vi "dioda.vi"() -> ()   [LabVIEW 2012]
panel:
  in  "data":bool[](array[boolean])
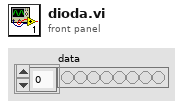
[diagram p1: front panel]
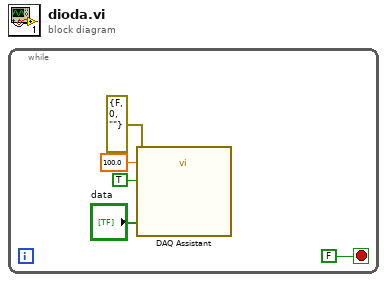
[diagram p0: block diagram]
diagram:
  n1 = while {
    stop <- FALSE stop-if-true
    n2 = call "DAQ Assistant"("data"="data", "timeout (s)"=100.0, "error in"=errorcluster {"status"=FALSE, "code"=0, "source"=""}, "stop (T)"=TRUE) -> ()  [unwired: 14 in, 2 out]
  }
